vi "FTW-Test-JSON-SpecialCharacters.vi"() -> ()   [LabVIEW 2018]
uses:
  dbc5f531-2408-43dc-9cfd-048e7de40848.vi
  3764b8bb-fed4-46cf-b0e2-6cf650a2cfe1.vi
  dbc5f531-2408-43dc-9cfd-048e7de40848.vi/4c6e0446-cc9c-4612-905b-49a825d4f3f2.vi
  source/container/FTW-Container-FromVariant.vi
  source/container/FTW-Container-New-FromContainer.vi
  source/JSON/FTW-JSON-SerializeAndDestroy.vi
  source/JSON/core/FTW-JSON-Core-EncodingFlags.vi
  source/Reflection/FTW-Reflection-Type.vi
  source/JSON/FTW-JSON-Parse.vi
  source/container/FTW-Container-GetFlattenedValue.vi
panel:
  out "String 3":string
  out "String 2":string
  in  "String":string="°"
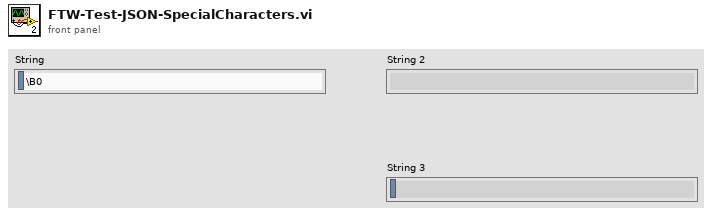
[diagram p1: front panel]
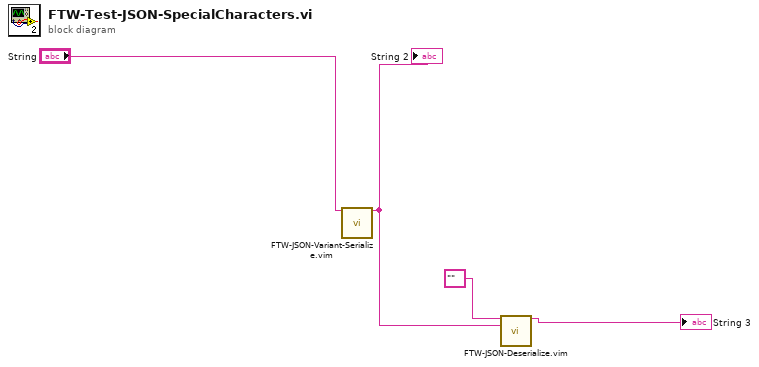
[diagram p0: block diagram]
diagram:
  n1 = call "FTW-JSON-Variant-Serialize.vim"("Variant"="String") -> ("JSON String"=w2:string)  [unwired: 13 in, 1 out]
  "String 2" <- w2
  n2 = call "FTW-JSON-Deserialize.vim"("Type In"="", "JSON String"=w2) -> ("Type Out"=→"String 3":string)  [unwired: 12 in, 1 out]
